vi "Write degreesAlt.vi"(8 "error in (no error)":errorcluster, 10 "degreesAlt":dbl[unit]=1.5707963267948966 min=0.08726646259971647 max=1.5707963267948966, 11 "Elevation in":refnum<class "Elevation.lvclass">) -> (0 "error out":errorcluster, 3 "Elevation out":refnum<class "Elevation.lvclass">)   [LabVIEW 2014, in "TCSDataDefinitions.lvlib" / "TCSCommand.lvlib" / "TargetConfiguration.lvlib" / "Target.lvlib" / "FixedTarget.lvlib" / "Elevation.lvclass"]
uses:
  Elevation.lvclass
  Elevation.lvclass/Elevation.ctl
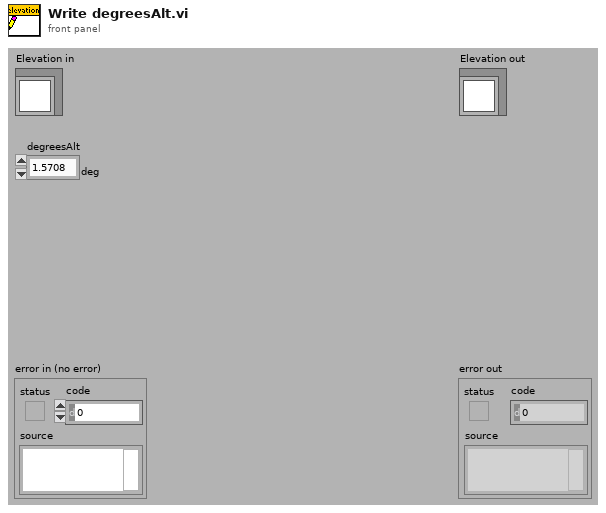
[diagram p1: front panel]
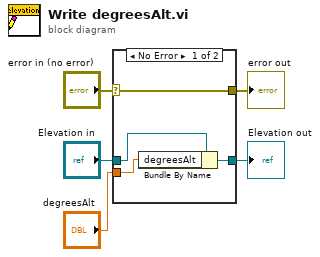
[diagram p0: block diagram]
diagram:
  n1 = case shown="No Error" "error in (no error)" {
    selector: "error in (no error)" -> [w9 w10]
    tunnel: [w9 w10] -> w4
    tunnel: [w7 w11] -> w2
    tunnel: "Elevation in" -> [w8 w11]
    tunnel: "degreesAlt" -> [w6 _]
    frame No Error {
      n2 = Bundle By Name(cluster=w8, "degreesAlt"=w6) -> (w7:refnum<class "Elevation.lvclass">)
    }
    frame Error {
    }
  }
  "error out" <- w4
  "Elevation out" <- w2
